vi "TCPSendSingleMulligan.vi"() -> ()   [LabVIEW 2013]
panel:
  out "Port Number":u16=50291
  in  "IP":string="128.8.195.108"
  out "Sent = Response":bool
  in  "File #":i32
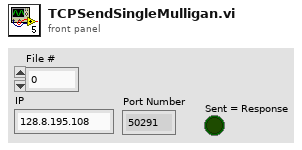
[diagram p1: front panel]
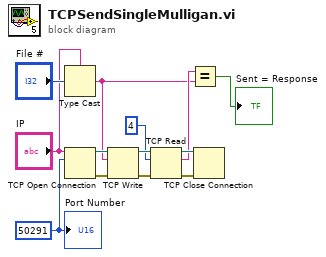
[diagram p0: block diagram]
diagram:
  w13 = u16 50291 ("remote port or service name")
  n1 = Type Cast(type="IP", x="File #") -> (*(type *) &x=w4:string)
  n2 = TCP Open Connection(address="IP", remote port or service name=w13) -> (connection ID=w11:refnum<k5>, error out=w12:errorcluster)  [unwired: 3 in]
  n3 = TCP Write(connection ID=w11, data in=w4, error in (no error)=w12) -> (connection ID out=w9:refnum<k5>, error out=w10:errorcluster)  [unwired: 1 in, 1 out]
  n4 = TCP Read(connection ID=w9, bytes to read=4, error in (no error)=w10) -> (connection ID out=w7:refnum<k5>, data out=w6:string, error out=w8:errorcluster)  [unwired: 2 in]
  n5 = Equal?(x=w6, y=w4) -> (x = y?=→"Sent = Response":bool)
  n6 = TCP Close Connection(connection ID=w7, error in (no error)=w8) -> ()  [unwired: 1 in, 2 out]
  "Port Number" <- w13
